vi "acender_led.vi"() -> ()   [LabVIEW 2018]
uses:
  <vilib>/Instr/_visa.llb/VISA Configure Serial Port (Instr).vi
panel:
  in  "stop":bool
  in  "OK Button":bool
  in  "VISA resource name":refnum<visa-resource-name>
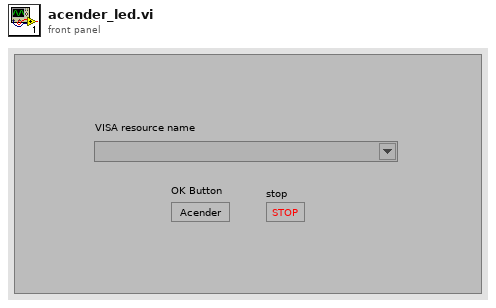
[diagram p1: front panel]
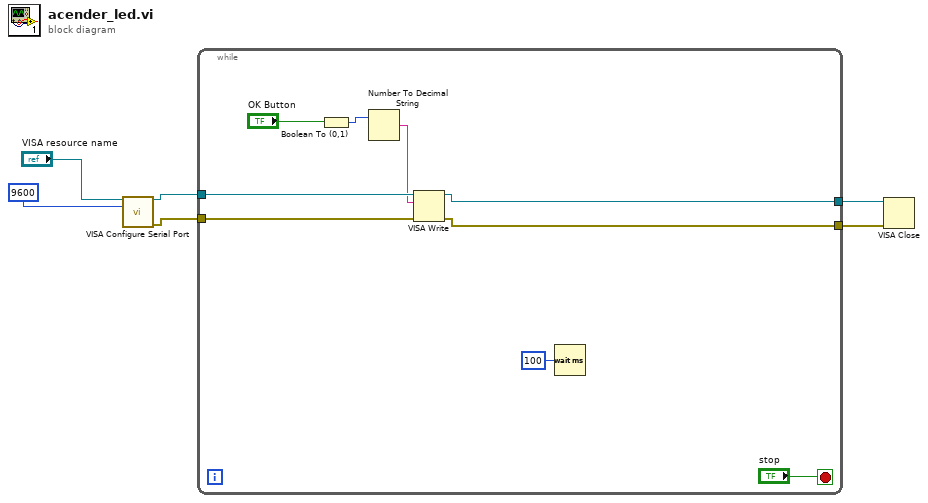
[diagram p0: block diagram]
diagram:
  n1 = call-poly "VISA Configure Serial Port"("VISA resource name"="VISA resource name", "baud rate (9600)"=u32 9600) -> ("VISA resource name out"=w4:refnum<visa-resource-name>, "error out"=w3:errorcluster)  [unwired: 12 in]
  n2 = while {
    tunnel: w4 -> [w15]
    tunnel: w3 -> [w14]
    tunnel: [w13] -> w2
    tunnel: [w12] -> w1
    stop <- "stop" stop-if-true
    n3 = Boolean To (0,1)(Boolean="OK Button") -> (0, 1=w8:i16)
    n4 = Number To Decimal String(number=w8) -> (decimal integer string=w7:string)  [unwired: 1 in]
    n5 = VISA Write(VISA resource name=w15, write buffer=w7, error in (no error)=w14) -> (VISA resource name out=w13:refnum<visa-resource-name>, error out=w12:errorcluster)  [unwired: 1 out]
    n6 = Wait (ms)(milliseconds to wait=u32 100) -> ()  [unwired: 1 out]
  }
  n7 = VISA Close(VISA resource name=w2, error in (no error)=w1) -> ()  [unwired: 1 out]
